vi "TestAccessibilty.vi"(8 "error in (no error)":errorcluster) -> (0 "error out":errorcluster)   [LabVIEW 2016, in "WeatherReportTests.lvlib"]
uses:
  WeatherReportTests.lvlib
  APIs/Stimulus/ControlValue/SetValueAuto.vi
  APIs/Stimulus/ControlValue/Controls/Tree/SetValueByHierarchicalPath.vi
  APIs/Stimulus/ControlValue/Controls/Listbox/SetValueByItemName.vi
  APIs/Assert/AssertControlProperty/AssertControlDisable/AssertEnabled.vi
  APIs/Assert/AssertControlProperty/AssertControlDisable/AssertDisabled.vi
  APIs/Assert/AssertControlProperty/AssertControlDisable/AssertDisabledAndGrayedOut.vi
  APIs/Stimulus/VI/CloseVI.vi
  Drona.lvlib
  <vilib>/addons/_JKI Toolkits/Caraya/classes/Test/Test.lvclass
  APIs/Stimulus/ControlValue/Controls/Listbox/StimulusListbox.lvlib
  APIs/Assert/AssertControlProperty/AssertControlDisable/AssertControlDisable.lvlib
  APIs/Stimulus/ControlValue/ControlValue.lvlib
  APIs/Stimulus/ControlValue/Controls/Tree/StimulusTree.lvlib
  APIs/Stimulus/VI/VI.lvlib
panel:
  # "Drona Test Accessibilty"
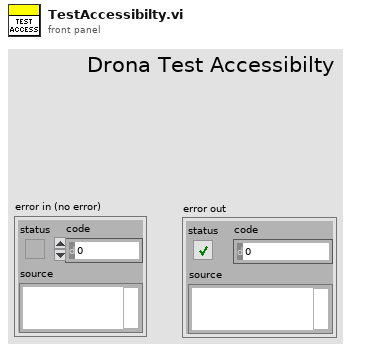
[diagram p1: front panel]
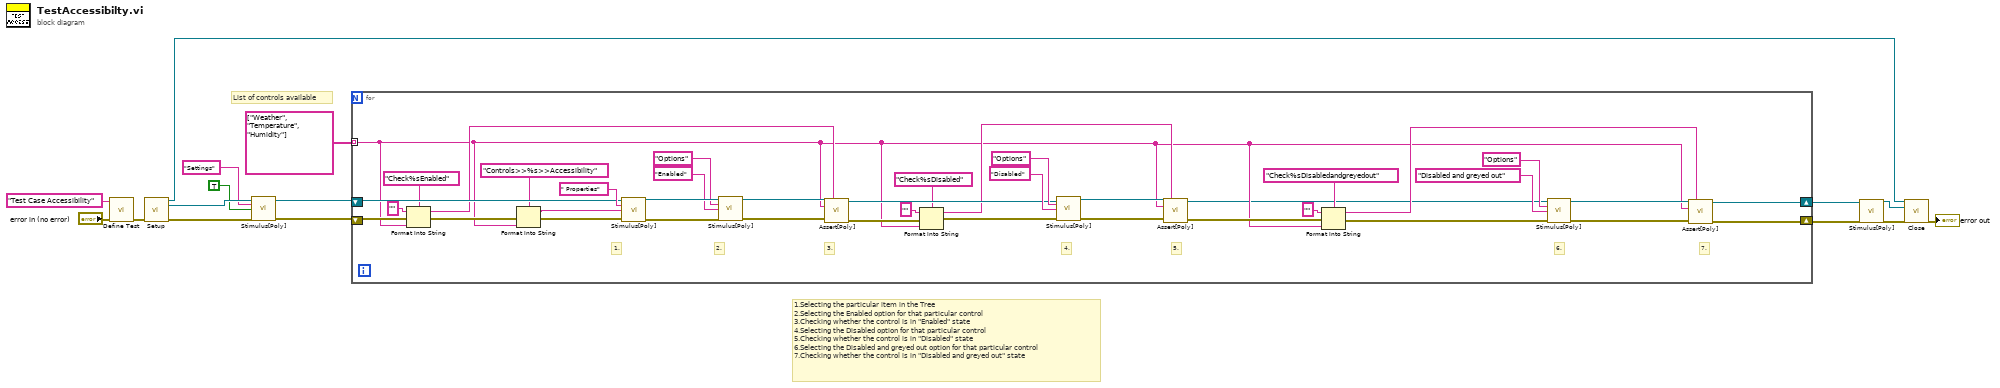
[diagram p0: block diagram]
diagram:
  # "1.Selecting the particular item in the Tree\n2.Selecting the Enabled option for that particular control\n3.Checking whether the control is in \"Enabled\" state\n4.Selecting the Disabled option for that particular control\n5.Checking whether the control is in \"Disabled\" state\n6.Selecting the Disabled and greyed out option for that particular control\n7.Checking whether the control is in \"Disabled and greyed out\" state"
  # "List of controls available"
  n1 = call <vilib>:"Define Test.vi"("error in (no error)"="error in (no error)", "Label (VI Title)"="Test Case Accessibility") -> ("error out"=w16:errorcluster)  [unwired: 8 in, 1 out]
  n2 = call "Setup.vi"("error in"=w16) -> ("Application Ref"=w7:refnum<vi>, "VI Reference Out"=w13:refnum<vi>, "error out"=w12:errorcluster)  [unwired: 12 in]
  n3 = call-poly "Stimulus[Poly].vi"("VI Reference In"=w13, "Control Path"="Settings", "Value (Signaling)"=TRUE, "error in"=w12) -> ("VI Reference Out"=w5:refnum<vi>, "error out"=w3:errorcluster)  [unwired: 10 in]
  n4 = for {
    tunnel: string[] ["Weather", "Temperature", "Humidity"] ("Control Path") -> [w19] mode=indexing
    shift-right: [w17] -> w2
    shift-left: w5 -> [w40]
    shift-right: [w38] -> w4
    shift-left: w3 -> [w34]
    # "7."
    # "6."
    # "5."
    # "4."
    # "3."
    # "2."
    # "1."
    n5 = Format Into String(format string="Check%sEnabled" ("Label"), initial string="", error in=w34, w19) -> (resulting string=w31:string, error out=w33:errorcluster)
    n6 = Format Into String(format string="Controls>>%s>>Accessibility" ("Control Path"), error in=w33, w19) -> (resulting string=w36:string, error out=w37:errorcluster)  [unwired: 1 in]
    n7 = call-poly "Stimulus[Poly].vi"("VI Reference In"=w40, "Control Path"=" Properties", "Hierarchical Path"=w36, "Error In"=w37) -> ("VI Reference Out"=w45:refnum<vi>, "Error Out"=w46:errorcluster)  [unwired: 10 in]
    n8 = call-poly "Stimulus[Poly].vi"("VI Reference In"=w45, "Control Path"="Options", "Item Name"="Enabled", "Error In"=w46) -> ("VI Reference Out"=w42:refnum<vi>, "Error Out"=w41:errorcluster)  [unwired: 10 in]
    n9 = call-poly "Assert[Poly].vi"("VI Reference In"=w42, "Test Label"=w31, "Control Path"=w19, "Error In"=w41) -> ("VI Reference Out"=w39:refnum<vi>, "Error Out"=w27:errorcluster)  [unwired: 9 in, 1 out]
    n10 = Format Into String(format string="Check%sDisabled" ("Label"), initial string="", error in=w27, w19) -> (resulting string=w25:string, error out=w26:errorcluster)
    n11 = call-poly "Stimulus[Poly].vi"("VI Reference In"=w39, "Control Path"="Options", "Item Name"="Disabled", "Error In"=w26) -> ("VI Reference Out"=w53:refnum<vi>, "Error Out"=w52:errorcluster)  [unwired: 10 in]
    n12 = call-poly "Assert[Poly].vi"("VI Reference In"=w53, "Test Label"=w25, "Control Path"=w19, "Error In"=w52) -> ("VI Reference Out"=w18:refnum<vi>, "Error Out"=w22:errorcluster)  [unwired: 9 in, 1 out]
    n13 = Format Into String(format string="Check%sDisabledandgreyedout" ("Label"), initial string="", error in=w22, w19) -> (resulting string=w20:string, error out=w21:errorcluster)
    n14 = call-poly "Stimulus[Poly].vi"("VI Reference In"=w18, "Control Path"="Options", "Item Name"="Disabled and greyed out", "Error In"=w21) -> ("VI Reference Out"=w50:refnum<vi>, "Error Out"=w51:errorcluster)  [unwired: 10 in]
    n15 = call-poly "Assert[Poly].vi"("VI Reference In"=w50, "Test Label"=w20, "Control Path"=w19, "Error In"=w51) -> ("VI Reference Out"=w17:refnum<vi>, "Error Out"=w38:errorcluster)  [unwired: 9 in, 1 out]
  }
  n16 = call-poly "Stimulus[Poly].vi"("VI Reference In"=w2, "error in"=w4) -> ("VI Reference Out"=w9:refnum<vi>, "error out"=w8:errorcluster)  [unwired: 12 in]
  n17 = call "Close.vi"("Application Ref"=w7, "VI Reference"=w9, "error in"=w8) -> ("error out"=→"error out":errorcluster)  [unwired: 12 in]
